vi "MCSGlobalVarsWrite.vi"(0 "MCSSelectTrigger":T2, 1 "delay(ticks)":u32, 2 "nOfBins":u32, 3 "nOfBunches":i32, 4 "MCSstate":T1, 10 "writeOnlyMCSState":bool) -> ()   [LabVIEW 2014]
uses:
  Controls/MCSselectTrigger.ctl
  Controls/MCSstate.ctl
  <vilib>/rvi/Emulation/niFpgaSctlEmulationGetInTimedLoop.vi
  MCSGlobalVars.vi
  <vilib>/rvi/Emulation/niFpgaProcessEmulError.vi
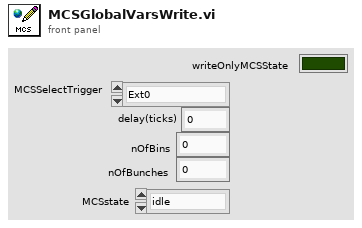
[diagram p1: front panel]
types:
  T1 = typedef "MCSstate.ctl" = enum16{"idle", "scanning", "done", "error"}
  T2 = typedef "MCSselectTrigger.ctl" = enum8{"Ext0", "Ext1", "Ext2", "Ext3", "Ext4", "Ext5", "Ext6", "Ext7", "Int0", "Int1", "Int2", "Int3", "Int4", "Int5", "Int6", "Int7"}
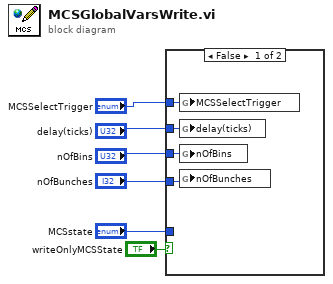
[diagram p0: block diagram]
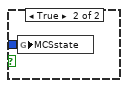
[diagram p2: hidden frame]
diagram:
  n1 = case shown="False" "writeOnlyMCSState" {
    tunnel: "MCSstate" -> [_ w11]
    tunnel: "MCSSelectTrigger" -> [w10 _]
    tunnel: "delay(ticks)" -> [w9 _]
    tunnel: "nOfBins" -> [w8 _]
    tunnel: "nOfBunches" -> [w7 _]
    frame False {
      n2 = global write "MCSGlobalVars.vi" "MCSSelectTrigger"(w10) -> ()
      n3 = global write "MCSGlobalVars.vi" "delay(ticks)"(w9) -> ()
      n4 = global write "MCSGlobalVars.vi" "nOfBins"(w8) -> ()
      n5 = global write "MCSGlobalVars.vi" "nOfBunches"(w7) -> ()
    }
    frame True {
      n6 = global write "MCSGlobalVars.vi" "MCSstate"(w11) -> ()
    }
  }
